vi "acquireData_2chan.vi"() -> ()   [LabVIEW 2023]
uses:
  <vilib>/DAQmx/read.llb/DAQmx Read (Analog 1D Wfm NChan NSamp).vi
  <vilib>/DAQmx/create/channels.llb/DAQmx Create Channel (AI-Voltage-Basic).vi
  <vilib>/DAQmx/configure/timing.llb/DAQmx Timing (Sample Clock).vi
  <vilib>/DAQmx/miscellaneous.llb/DAQmx Fill In Error Info.vi
  <resource>/objmgr/daqmx.rc
panel:
  out "data":waveform(dbl)[](array[waveform])
  in  "AI Channel 2 Name":string="/ai2"
  out "Waveform Graph":waveform(dbl)[](graph)
  in  "Play Measured Signal?":bool
  in  "AI Channel 1 Name":string="/ai1"
  out "error out":errorcluster
  in  "Sampling Rate":dbl
  in  "Receive Duration":dbl
  in  "DAQmx Device Name":tag
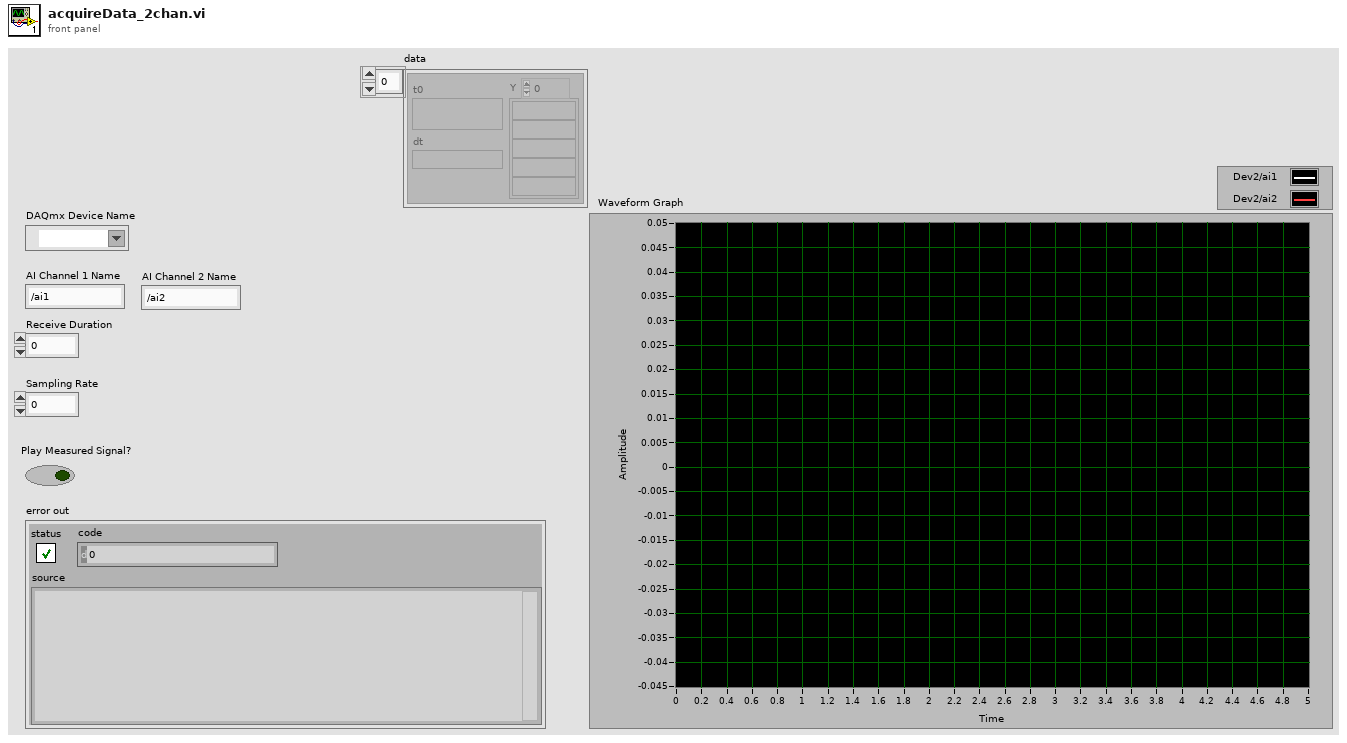
[diagram p1: front panel]
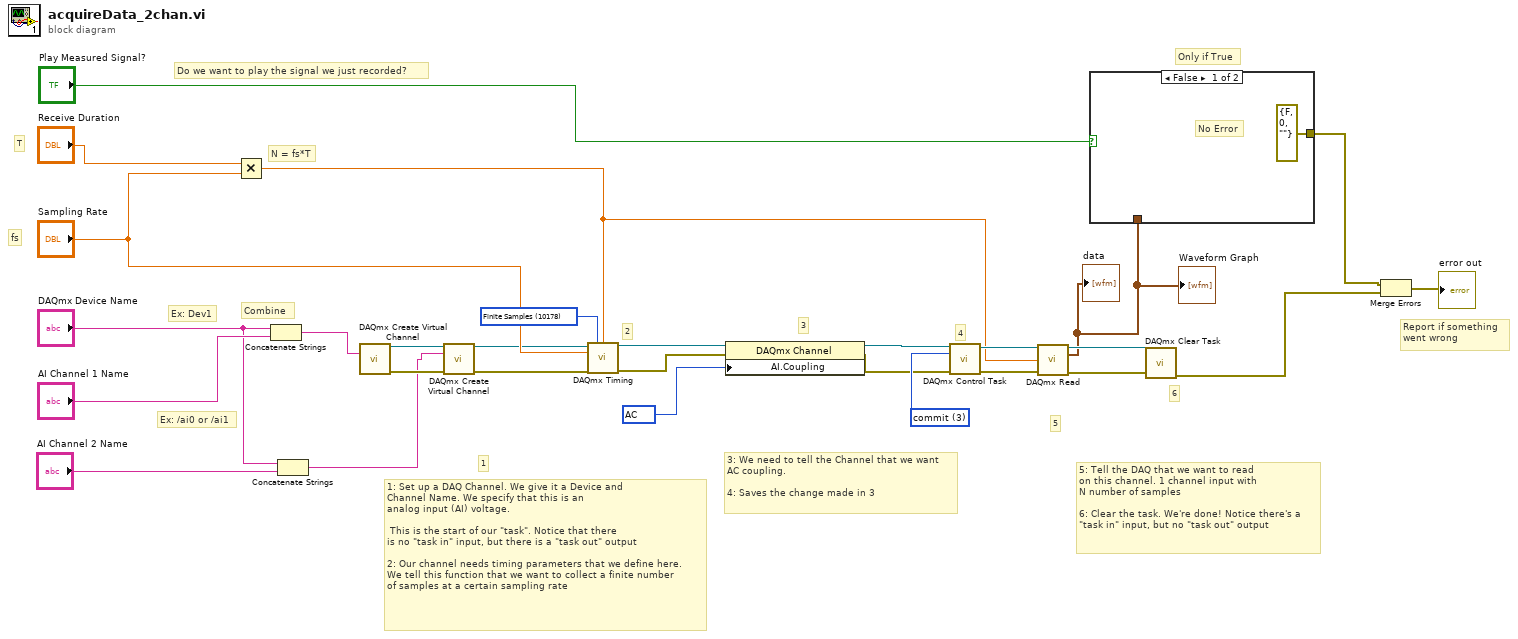
[diagram p0: block diagram]
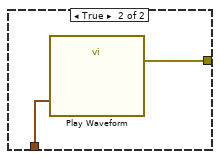
[diagram p2: hidden frame]
diagram:
  w26 = 10045 items=["AC"=10045, "DC"=10050, "GND"=10066] ("AI.Coupling")
  w27 = 10178 items=["Finite Samples"=10178, "Continuous Samples"=10123, "Hardware Timed Single Point"=12522] ("sample mode")
  w28 = 3 items=["verify"=2, "reserve"=4, "commit"=3, "unreserve"=5, "abort"=6] ("action")
  # "Only if True"
  # "5: Tell the DAQ that we want to read\non this channel. 1 channel input with\nN number of samples\n\n6: Clear the task. We're done! Notice there's a \n\"task in\" input, but no \"task out\" output"
  # "Report if something\nwent wrong"
  # "Do we want to play the signal we just recorded?"
  # "6"
  # "5"
  # "3: We need to tell the Channel that we want\nAC coupling.\n\n4: Saves the change made in 3"
  # "1: Set up a DAQ Channel. We give it a Device and \nChannel Name. We specify that this is an \nanalog input (AI) voltage.\n\n This is the start of our \"task\". Notice that there\nis no \"task in\" input, but there is a \"task out\" output\n\n2: Our channel needs timing parameters that we define here.\nWe tell this function that we want to collect a finite number\nof samples at a certain sampling rate"
  # "4"
  # "3"
  # "2"
  # "1"
  # "Ex: Dev1"
  # "Ex: /ai0 or /ai1"
  # "Combine"
  # "N = fs*T"
  # "T"
  # "fs"
  n1 = Multiply(x="Receive Duration", y="Sampling Rate") -> (x*y=w16:dbl)
  n2 = Concatenate Strings("DAQmx Device Name", "AI Channel 1 Name") -> (w2:string)
  n3 = Concatenate Strings("DAQmx Device Name", "AI Channel 2 Name") -> (w1:string)
  n4 = call-poly <vilib>:"DAQmx Create Virtual Channel.vi"("physical channels"=w2) -> ("task out"=w8:refnum<k21>, "error out"=w6:errorcluster)  [unwired: 13 in]
  n5 = call-poly <vilib>:"DAQmx Create Virtual Channel.vi"("task in"=w8, "physical channels"=w1, "error in"=w6) -> ("task out"=w7:refnum<k21>, "error out"=w5:errorcluster)  [unwired: 11 in]
  n6 = call-poly <vilib>:"DAQmx Timing.vi"("task/channels in"=w7, "sample mode"=w27, "samples per channel"=w16, "rate"="Sampling Rate", "error in"=w5) -> ("task out"=w25:refnum<k21>, "error out"=w24:errorcluster)  [unwired: 9 in]
  n7 = property class="DAQmx Channel"(reference=w25, error in=w24, "AI.Coupling"=w26) -> (reference out=w23:refnum<k21>, error out=w22:errorcluster)
  n8 = call <vilib>:"DAQmx Control Task.vi"("task/channels in"=w23, "action"=w28, "error in"=w22) -> ("task out"=w21:refnum<k21>, "error out"=w20:errorcluster)  [unwired: 11 in]
  n9 = call-poly <vilib>:"DAQmx Read.vi"("task/channels in"=w21, "number of samples per channel"=w16, "error in"=w20) -> ("task out"=w19:refnum<k21>, "data"=w9:waveform(dbl)[], "error out"=w18:errorcluster)  [unwired: 10 in]
  "Waveform Graph" <- w9
  "data" <- w9
  n10 = case shown="False" "Play Measured Signal?" {
    tunnel: w9 -> [_ w31]
    tunnel: [errorcluster {"status"=FALSE, "code"=0, "source"=""} ("error out") w30] -> w11
    frame False {
      # "No Error"
    }
    frame True {
      n11 = call "Play Waveform"("Data"=w31) -> ("error out"=w30:errorcluster)  [unwired: 18 in]
    }
  }
  n12 = call <vilib>:"DAQmx Clear Task.vi"("task in"=w19, "error in"=w18) -> ("error out"=w12:errorcluster)  [unwired: 13 in]
  n13 = Merge Errors(w11, w12) -> (→"error out":errorcluster)
